vi "Read two switches.vi"(4 "Error In":errorcluster, 5 "LS2 Pin":u8, 6 "LS1 Pin":u8, 7 "LINX Resource":T1) -> (0 "Error Out":errorcluster, 1 "LS2 Value":bool, 2 "LS1 Value":bool, 3 "LINX Resource 2":T1)   [LabVIEW 2015]
uses:
  <vilib>/MakerHub/LINX/Private/Type Defs/LINX Ref.ctl
  <vilib>/MakerHub/LINX/Private/Type Defs/Platform.ctl
  <vilib>/MakerHub/LINX/Private/Type Defs/Interface.ctl
  <vilib>/MakerHub/LINX/Private/Device/Type Defs/LINX Device Config.ctl
  <vilib>/MakerHub/LINX/Private/Device/Type Defs/TCP Config.ctl
  <vilib>/MakerHub/LINX/Private/Device/Type Defs/Channels.ctl
  <vilib>/MakerHub/LINX/Public/Peripherals/Digital/Digital Read 1 Chan.vi
  <vilib>/MakerHub/LINX/LMH-LINX.lvlib
  <vilib>/MakerHub/LINX/Private/Device/Device.lvlib
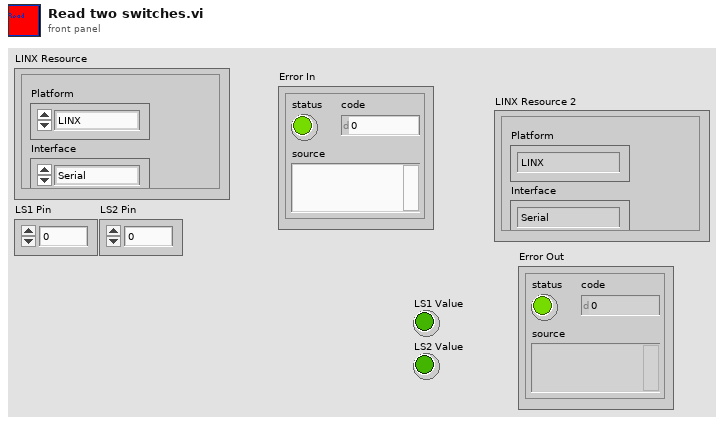
[diagram p1: front panel]
types:
  T1 = typedef "LMH-LINX.lvlib/LINX Ref.ctl" = cluster{"Platform":T2, "Interface":T3, "LINX Device Config":T4}
  T2 = typedef "LMH-LINX.lvlib/Platform.ctl" = enum16{"LINX", "myRIO"}
  T3 = typedef "LMH-LINX.lvlib/Interface.ctl" = enum16{"Serial", "TCP"}
  T4 = typedef "LMH-LINX.lvlib/Device.lvlib/LINX Device Config.ctl" = cluster{"Interface":T3, "COM Port":refnum<visa-resource-name>, "TCP Configuration":T5, "Device Family":u8, "Device ID":u8, "Device Name":string, "TCP Ref":refnum<k5>, "Channels":T6}
  T5 = typedef "LMH-LINX.lvlib/Device.lvlib/TCP Config.ctl" = cluster{"IP Address":string, "Port":u16}
  T6 = typedef "LMH-LINX.lvlib/Channels.ctl" = cluster{"DI":u8[], "DO":u8[], "AI":u8[], "AO":u8[], "PWM":u8[], "QE":u8[], "UART":u8[], "I2C 2":u8[], "SPI":u8[], "CAN":u8[], "Servo":u8[], "AI Ref (V)":dbl, "AO Ref (V)":dbl, "AO Resolution (Bits)":u8}
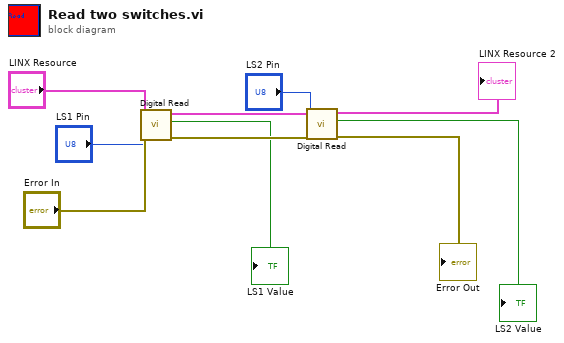
[diagram p0: block diagram]
diagram:
  n1 = call-poly <vilib>:"Digital Read.vi"("Error In"="Error In", "DI Channel"="LS1 Pin", "LINX Resource"="LINX Resource") -> ("Error Out"=w6:errorcluster, "DI Value"=→"LS1 Value":bool, "LINX Resource"=w7:T1)  [unwired: 6 in]
  n2 = call-poly <vilib>:"Digital Read.vi"("Error In"=w6, "DI Channel"="LS2 Pin", "LINX Resource"=w7) -> ("Error Out"=→"Error Out":errorcluster, "DI Value"=→"LS2 Value":bool, "LINX Resource"=→"LINX Resource 2":T1)  [unwired: 6 in]
